vi "GETPORTSTATUS.vi"(8 "error in (no error)":errorcluster, 10 "Port to read":dbl, 11 "simulado in":refnum<class "simulado.lvclass">) -> (0 "error out":errorcluster, 3 "simulado out":refnum<class "simulado.lvclass">)   [LabVIEW 2019, in "simulado.lvclass"]
uses:
  simulado.lvclass
  simulado.lvclass/simulado.ctl
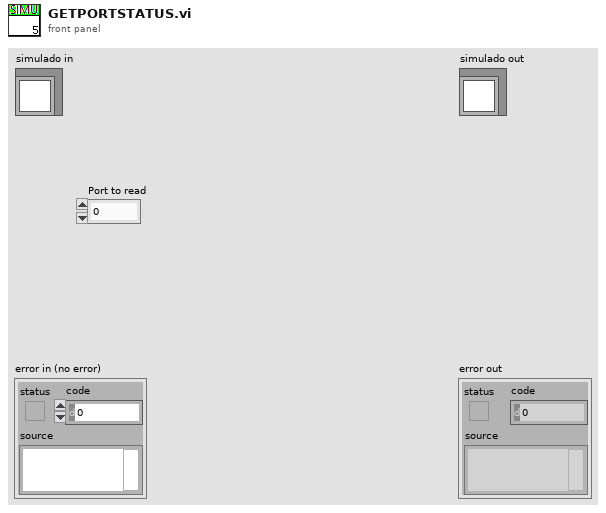
[diagram p1: front panel]
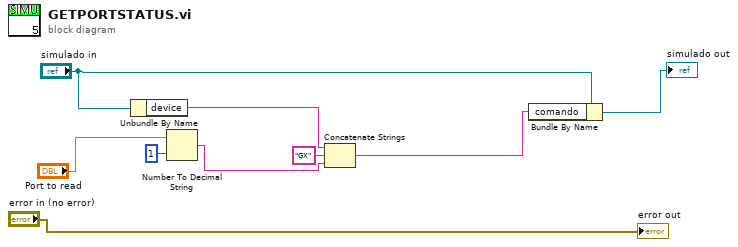
[diagram p0: block diagram]
diagram:
  n1 = Unbundle By Name("simulado in") -> ("device"=w5:string)
  n2 = Number To Decimal String(number="Port to read", width (-)=i16 1) -> (decimal integer string=w3:string)
  n3 = Concatenate Strings(w5, "GX" ("string"), w3) -> (w1:string)
  n4 = Bundle By Name(cluster="simulado in", "comando"=w1) -> (→"simulado out":refnum<class "simulado.lvclass">)
  "error out" <- "error in (no error)"
